vi "forward.vi"(9 "RobotParams":T1={"R1"=31.0, "R2"=37.0, "R3"=31.0, "RadsPerCnt"=0.0, "EncOffset1"=0, "EncOffset2"=0, "HomeX"=0.0, "HomeY"=0.0}, 10 "Enc 2":i32, 11 "Enc 1":i32) -> (0 "Y raw":dbl, 1 "Y":dbl, 2 "X":dbl, 3 "X raw":dbl, 4 "Jt":dbl[][](array[numeric]))   [LabVIEW 2019]
uses:
  RobotParams.ctl
  <vilib>/imath/engines/lvmath2/RunTimeEngine/IndexReplace/NIMS V(S)=S.vi
  <instcachedir>/0/NIMS V(S)=S_BD5C8CB81B6E4D99B8C0034EA1BEE55D.lvgen/NIMS V(S)=S_BD5C8CB81B6E4D99B8C0034EA1BEE55D_000.vi
  <vilib>/imathl/engines/lvmath/Functions/Error Handling/Create Error.vi
  <vilib>/imath/engines/lvmath2/RunTimeEngine/IndexRead/NIMS V(S).vi
  <instcachedir>/0/NIMS V(S)_0488751826AF41519A22953C041130DC.lvgen/NIMS V(S)_0488751826AF41519A22953C041130DC_000.vi
  <vilib>/imath/engines/lvmath2/RunTimeEngine/NodeEndStatement/NIMS_NodeEndStatement_Output.vi
  <instcachedir>/0/NIMS_NodeEndStatement_Output_53EC0D466D134D7ABD903AC30B43404B.lvgen/NIMS_NodeEndStatement_Output_53EC0D466D134D7ABD903AC30B43404B_003.vi
  <instcachedir>/0/NIMS_NodeEndStatement_Output_53EC0D466D134D7ABD903AC30B43404B.lvgen/NIMS_NodeEndStatement_Output_53EC0D466D134D7ABD903AC30B43404B_009.vi
  <vilib>/imath/engines/lvmath2/RunTimeEngine/ErrorHandling/NIMS_Finalize Error.vi
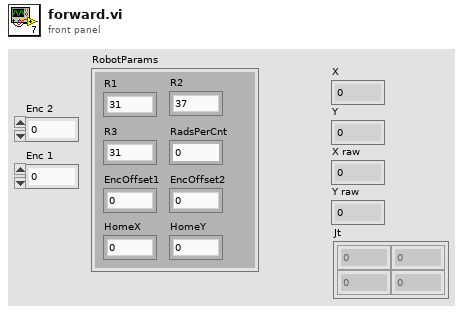
[diagram p1: front panel]
types:
  T1 = typedef "RobotParams.ctl" = cluster{"R1":dbl, "R2":dbl, "R3":dbl, "RadsPerCnt":dbl, "EncOffset1":i32, "EncOffset2":i32, "HomeX":dbl, "HomeY":dbl}
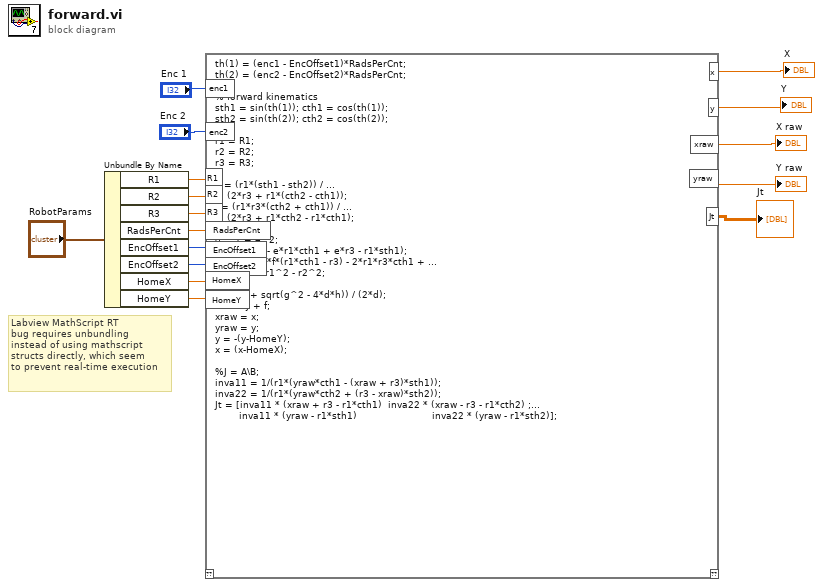
[diagram p0: block diagram]
diagram:
  # "Labview MathScript RT\nbug requires unbundling\ninstead of using mathscript\nstructs directly, which seem\nto prevent real-time execution"
  n1 = Unbundle By Name("RobotParams") -> ("R1"=w8:dbl, "R2"=w7:dbl, "R3"=w6:dbl, "RadsPerCnt"=w5:dbl, "EncOffset1"=w4:i32, "EncOffset2"=w3:i32, "HomeX"=w2:dbl, "HomeY"=w1:dbl)
  n2 = mathscript code="th(1) = (enc1 - EncOffset1)*RadsPerCnt;\nth(2) = (enc2 - EncOffset2)*RadsPerCnt;\n\n% forward kinematics\nsth1 = sin(th(1)); cth1 = cos(th(1));\nsth2 = sin(th(2)); cth2 = cos(th(2));\n\nr1 = R1;\nr2 = R2;\nr3 = R3;\n\ne = (r1*(sth1 - sth2)) / ...\n    (2*r3 + r1*(cth2 - cth1));\nf = (r1*r3*(cth2 + cth1)) / ...\n    (2*r3 + r1*cth2 - r1*cth1);\n\nd = 1 + e^2;\ng = 2*(e*f - e*r1*cth1 + e*r3 - r1*sth1);\nh = f^2 - 2*f*(r1*cth1 - r3) - 2*r1*r3*cth1 + ...\n    r3^2 + r1^2 - r2^2;\n\ny = (-g + sqrt(g^2 - 4*d*h)) / (2*d);\nx = e*y + f;\nxraw = x;\nyraw = y;\ny = -(y-HomeY);\nx = (x-HomeX);\n\n%J = A\\B;\ninva11 = 1/(r1*(yraw*cth1 - (xraw + r3)*sth1)); \ninva22 = 1/(r1*(yraw*cth2 + (r3 - xraw)*sth2));\nJt = [inva11 * (xraw + r3 - r1*cth1)\t\tinva22 * (xraw - r3 - r1*cth2) ;...\n     \t  inva11 * (yraw - r1*sth1)\t\t\t                      inva22 * (yraw - r1*sth2)];"("enc1"="Enc 1", "enc2"="Enc 2", "R1"=w8, "R2"=w7, "R3"=w6, "RadsPerCnt"=w5, "EncOffset1"=w4, "EncOffset2"=w3, "HomeX"=w2, "HomeY"=w1) -> ("x"=→"X":cdb, "y"=→"Y":cdb, "xraw"=→"X raw":cdb, "yraw"=→"Y raw":cdb, "Jt"=→"Jt":cdb[][])  [unwired: 1 in, 1 out]
